vi "Teleop.vi"(10 "Match Info":T1={"Autonomous Elapsed Seconds"=0.0, "TeleOp Elapsed Seconds"=0.0, "Disabled Elapsed Seconds"=0.0, "Visited Autonomous"=FALSE, "Visited TeleOp"=FALSE, "Visited Disabled"=FALSE, "Autonomous Settings"={"Autonomous Style"=enum."Independent", "VI Refnum"=refnum}}, 11 "Call Context":T2) -> ()   [LabVIEW 2012]
doc: "This VI is called for each TeleOp packet received from the DS where the robot is not disabled. It is often used to read from the joysticks and update I/O or to update setpoints for timed control loops. It should complete and return within 20 milliseconds or it may miss DS packets."
uses:
  <vilib>/Rock Robotics/WPI/DriverStation/WPI_DriverStationDerivedRobotMode.ctl
  <vilib>/Rock Robotics/WPI/DriverStation/WPI_DriverStationMatch Info.ctl
  RefnameEnum.ctl
  Robot Global Data.vi
  <vilib>/Rock Robotics/WPI/Joystick/WPI_JoystickGetSetRefNum.vi
  State_Machine_Enum.ctl
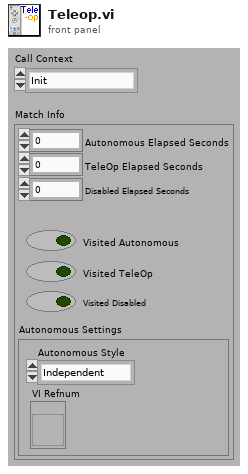
[diagram p1: front panel]
types:
  T1 = typedef "WPI_DriverStationMatch Info.ctl" = cluster{"Autonomous Elapsed Seconds":dbl, "TeleOp Elapsed Seconds":dbl, "Disabled Elapsed Seconds":dbl, "Visited Autonomous":bool, "Visited TeleOp":bool, "Visited Disabled":bool, "Autonomous Settings":cluster{"Autonomous Style":enum16{"Iterative", "Independent"}, "VI Refnum":refnum<vi>}}
  T2 = typedef "WPI_DriverStationDerivedRobotMode.ctl" = enum16{"Init", "Execute", "Stop"}
  T3 = typedef "State_Machine_Enum.ctl" = enum16{"Idle", "Start", "Do", "Stop", "Init"}
  T4 = typedef "RefnameEnum.ctl" = enum16{"FireLauncher", "Climber", "Shield", "TankDrive", "DriveEncoderL", "DriveEncoderR", "LauncherMotorRPM", "LauncherEncoderAnalog", "LauncherEncoderRPM", "ShooterLS", "DriveAlignLSLeft", "DriveAlignLSRight", "ClimbingLS", "LauncherEncoderAngle", "LauncherMotorAngle", "Gamepad1", "Gamepad2", "Compressor", "ClimbWeightSol3", "ClimbWeightSol4"}
  T5 = typedef "WPI_JoystickDevRef.ctl" = cluster{"Device":T6}
  T6 = typedef "WPI_JoystickDeviceEnum.ctl" = enum16{"USB 1", "USB 2", "USB 3", "USB 4", "Kinect 1", "Kinect 2"}
  T7 = typedef "WPI_JoystickButtonState.ctl" = cluster{"Button 1":bool, "Button 2":bool, "Button 3":bool, "Button 4":bool, "Button 5":bool, "Button 6":bool, "Button 7":bool, "Button 8":bool, "Button 9":bool, "Button 10":bool, "Button 11":bool, "Button 12":bool}
  T8 = cluster{"axis 1 (x)":dbl, "axis 2 (y)":dbl, "axis 3 (throttle)":dbl, "axis 4":dbl, "axis 5":dbl, "axis 6":dbl}
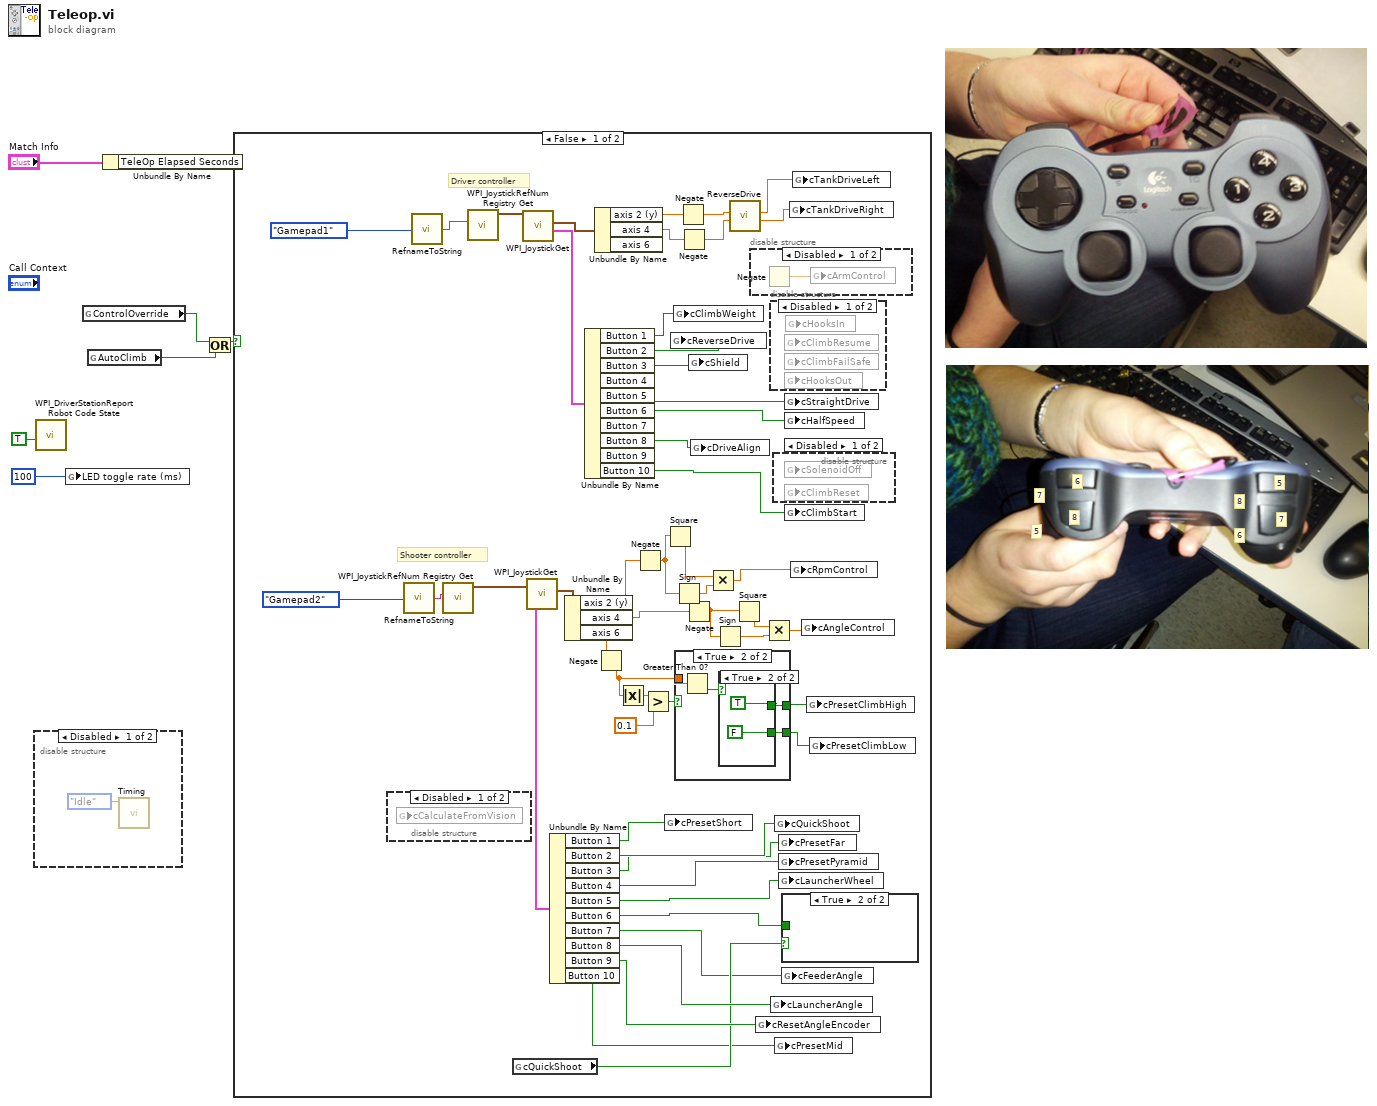
[diagram p0: block diagram]
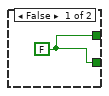
[diagram p3: hidden frame]
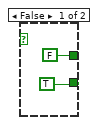
[diagram p4: hidden frame]
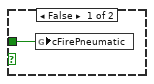
[diagram p5: hidden frame]
diagram:
  # "5"
  # "7"
  # "6"
  # "8"
  # "8"
  # "7"
  # "6"
  # "5"
  n1 = disable-structure shown="Disabled" {
    frame Disabled {
      n2 = call "Timing.vi"("State"=State_Machine_Enum."Idle") -> ()  [unwired: 9 in, 2 out]
    }
    frame Enabled {
    }
  }
  n3 = call <vilib>:"WPI_DriverStationReport Robot Code State.vi"("TeleOp"=TRUE ("Autonomous")) -> ()  [unwired: 10 in, 1 out]
  n4 = global write "Robot Global Data.vi" "LED toggle rate (ms)"(u32 100 ("LED ms toggle rate")) -> ()
  n5 = global read "Robot Global Data.vi" "ControlOverride"() -> (w3:bool)
  n6 = global read "Robot Global Data.vi" "AutoClimb"() -> (w1:bool)
  n7 = Unbundle By Name("Match Info") -> ()  [unwired: 1 out]
  n8 = Or(x=w3, y=w1) -> (x .or. y?=w2:bool)
  n9 = case shown="False" w2 {
    frame False {
      # "Shooter controller"
      # "Driver controller"
      n10 = disable-structure shown="Disabled" {
        frame Disabled {
          n11 = global read "Robot Global Data.vi" "cCalculateFromVision"() -> ()  [unwired: 1 in]
        }
        frame Enabled {
        }
      }
      n12 = call "RefnameToString.vi"("Enum"=RefnameEnum."Gamepad2") -> ("Refname"=w19:string)
      n13 = call "RefnameToString.vi"("Enum"=RefnameEnum."Gamepad1") -> ("Refname"=w21:string)
      n14 = call <vilib>:"WPI_JoystickRefNum Registry Get.vi"("refnum name"=w19) -> ("JoystickDevRef"=w57:T5)  [unwired: 1 in, 9 out]
      n15 = call <vilib>:"WPI_JoystickRefNum Registry Get.vi"("refnum name"=w21) -> ("JoystickDevRef"=w58:T5)  [unwired: 1 in, 9 out]
      n16 = global read "Robot Global Data.vi" "cQuickShoot"() -> (w23:bool)
      n17 = call <vilib>:"WPI_JoystickGet.vi"("JoystickDevRef"=w58) -> ("Buttons"=w54:T7, "Axes"=w56:T8)  [unwired: 4 in, 1 out]
      n18 = call <vilib>:"WPI_JoystickGet.vi"("JoystickDevRef"=w57) -> ("Buttons"=w52:T7, "Axes"=w53:T8)  [unwired: 4 in, 1 out]
      n19 = Unbundle By Name(w52) -> ("Button 1"=w17:bool, "Button 2"=w51:bool, "Button 3"=w50:bool, "Button 4"=w49:bool, "Button 5"=w48:bool, "Button 6"=w47:bool, "Button 7"=w18:bool, "Button 8"=w37:bool, "Button 9"=w25:bool, "Button 10"=w16:bool)
      n20 = Unbundle By Name(w53) -> ("axis 2 (y)"=w44:dbl, "axis 4"=w42:dbl, "axis 6"=w15:dbl)
      n21 = Unbundle By Name(w54) -> ("Button 1"=w9:bool, "Button 2"=w24:bool, "Button 3"=w32:bool, "Button 5"=w40:bool, "Button 6"=w38:bool, "Button 8"=w26:bool, "Button 10"=w39:bool)  [unwired: 3 out]
      n22 = Unbundle By Name(w56) -> ("axis 2 (y)"=w55:dbl, "axis 4"=w30:dbl)  [unwired: 1 out]
      n23 = Negate(x=w15) -> (-x=w8:dbl)
      n24 = Absolute Value(x=w8) -> (abs(x)=w14:dbl)
      n25 = Negate(x=w44) -> (-x=w34:dbl)
      n26 = Greater?(x=w14, y=0.1) -> (0:w13:bool)
      n27 = Square(x=w34) -> (x^2=w46:dbl)
      n28 = global write "Robot Global Data.vi" "cPresetShort"(w17) -> ()
      n29 = global write "Robot Global Data.vi" "cReverseDrive"(w24) -> ()
      n30 = global write "Robot Global Data.vi" "cClimbWeight"(w9) -> ()
      n31 = Sign(1:w34) -> (0:w45:dbl)
      n32 = case shown="True" w13 {
        tunnel: w8 -> [_ w62]
        tunnel: [w59 w61] -> w11
        tunnel: [w59 w60] -> w10
        frame False {
          w59 = FALSE
        }
        frame True {
          n33 = Greater Than 0?(x=w62) -> (x > 0?=w63:bool)
          n34 = case shown="True" w63 {
            tunnel: [FALSE TRUE] -> w61
            tunnel: [TRUE FALSE] -> w60
            frame False {
            }
            frame True {
            }
          }
        }
      }
      n35 = Negate(x=w55) -> (-x=w31:dbl)
      n36 = Negate(x=w30) -> (-x=w29:dbl)
      n37 = Negate(x=w42) -> (-x=w33:dbl)
      n38 = global write "Robot Global Data.vi" "cShield"(w32) -> ()
      n39 = global write "Robot Global Data.vi" "cDriveAlign"(w26) -> ()
      n40 = Multiply(x=w46, y=w45) -> (x*y=w36:dbl)
      n41 = Sign(1:w33) -> (0:w43:dbl)
      n42 = call "ReverseDrive.vi"("InitLeft"=w31, "InitRight"=w29) -> ("Final Left"=w28:dbl, "FinalRight"=w27:dbl)  [unwired: 7 in]
      n43 = Square(x=w33) -> (x^2=w41:dbl)
      n44 = disable-structure shown="Disabled" {
        frame Disabled {
          n45 = Negate() -> (-x=w69:dbl)  [unwired: 1 in]
          n46 = global write "Robot Global Data.vi" "cArmControl"(w69) -> ()
        }
        frame Enabled {
        }
      }
      n47 = global write "Robot Global Data.vi" "cResetAngleEncoder"(w25) -> ()
      n48 = Multiply(x=w41, y=w43) -> (x*y=w35:dbl)
      n49 = disable-structure shown="Disabled" {
        frame Disabled {
          n50 = global read "Robot Global Data.vi" "cClimbResume"() -> ()  [unwired: 1 in]
          n51 = global read "Robot Global Data.vi" "cClimbFailSafe"() -> ()  [unwired: 1 in]
          n52 = global read "Robot Global Data.vi" "cHooksOut"() -> ()  [unwired: 1 in]
          n53 = global read "Robot Global Data.vi" "cHooksIn"() -> ()  [unwired: 1 in]
        }
        frame Enabled {
        }
      }
      n54 = global write "Robot Global Data.vi" "cLauncherAngle"(w37) -> ()
      n55 = disable-structure shown="Disabled" {
        frame Disabled {
          n56 = global read "Robot Global Data.vi" "cSolenoidOff"() -> ()  [unwired: 1 in]
          n57 = global read "Robot Global Data.vi" "cClimbReset"() -> ()  [unwired: 1 in]
        }
        frame Enabled {
        }
      }
      n58 = global write "Robot Global Data.vi" "cQuickShoot"(w51) -> ()
      n59 = global write "Robot Global Data.vi" "cPresetMid"(w16) -> ()
      n60 = global write "Robot Global Data.vi" "cPresetFar"(w50) -> ()
      n61 = global write "Robot Global Data.vi" "cPresetPyramid"(w49) -> ()
      n62 = global write "Robot Global Data.vi" "cLauncherWheel"(w48) -> ()
      n63 = case shown="True" w23 {
        tunnel: w47 -> [w68 _]
        frame False {
          n64 = global write "Robot Global Data.vi" "cFirePneumatic"(w68) -> ()
        }
        frame True {
        }
      }
      n65 = global write "Robot Global Data.vi" "cFeederAngle"(w18) -> ()
      n66 = global write "Robot Global Data.vi" "cStraightDrive"(w40) -> ()
      n67 = global write "Robot Global Data.vi" "cHalfSpeed"(w38) -> ()
      n68 = global write "Robot Global Data.vi" "cClimbStart"(w39) -> ()
      n69 = global write "Robot Global Data.vi" "cTankDriveRight"(w27) -> ()
      n70 = global write "Robot Global Data.vi" "cRpmControl"(w36) -> ()
      n71 = global write "Robot Global Data.vi" "cTankDriveLeft"(w28) -> ()
      n72 = global write "Robot Global Data.vi" "cAngleControl"(w35) -> ()
      n73 = global write "Robot Global Data.vi" "cPresetClimbHigh"(w11) -> ()
      n74 = global write "Robot Global Data.vi" "cPresetClimbLow"(w10) -> ()
    }
    frame True {
    }
  }
